vi "NewIndependentStage.vi"() -> ()   [LabVIEW 2020]
uses:
  StageOptions.ctl
  SettingCtrlOptions.ctl
  PosCtrlOptions.ctl
  libximc.lvlib
  <instrlib>/_niInstr/Basic Elements/v1/FPGA/niInstr Basic Elements v1 FPGA.lvlib
panel:
  out "Y Maximum":dbl=220.0
  out "X Max Stage":dbl=220.0 format="%#_13g"
  out "Move Step halved":dbl=1.0
  in  "Next Coordinate Index":i32
  out "Step Sizes":sgl[](array[numeric])
  out "IDs":i32[](array[numeric])
  out "Calibration":cluster{dbl, "MicrostepMode":u32}[](array[cluster])
  out "Serial nos":u32[](array[numeric])
  in  "EdgePt/nPixelMap":bool=TRUE
  out "Stage Status":T1
  in  "Machine Mode":T2(ring)=enum."Normal"
  in  "Close Stage":bool
  in  "Move Step":dbl=1.0
  in  "Start Stage":bool
  in  "Speed Control (mm/s)":sgl(slide)=1.0 min=0.1 scale=0.1..5.0
  out "Y Step Size":sgl format="%#_2g"
  out "X Step Size":sgl format="%#_2g"
  in  "Scan Mode":enum16{"Raster", "Serpentine"}(ring)
  out "Controller Open?":bool
  in  "Y Position Abs":dbl caption="Y Position"
  in  "X Position Abs":dbl caption="X Position"
  in  "Move to Start":bool
  in  "Stop Stage":bool
  in  "Outline":bool
  in  "Stop Motion":bool
  in  "Right":bool
  in  "Left":bool
  in  "Down":bool
  in  "Up":bool
  in  "AbsMove":bool
  out "Moving?":bool
  in  "Zero":bool
  out "Y Position":dbl format="%#.3g"
  out "X Position":dbl format="%#.3g"
  out "Stage Position":cluster{sgl[], sgl[]}(graph) caption="XY Graph - Dark"
  in  "X Start":sgl
  in  "X End":sgl=10.0
  in  "Y Start":sgl
  in  "Y End":sgl=8.0
  in  "Y Step Size":sgl=0.5
  in  "X Step Size":sgl=0.5
  out "Line Count":i32=6
  out "Pixel Count":i32=6
  out "Peripheral Coordis":sgl[][](array[numeric])=[[0.0, 0.0], [1.8, 0.0], [3.6, 0.0], [5.3999996, 0.0], [7.2, 0.0], [9.0, 0.0], [9.0, 2.0], [7.2, 2.0], [5.3999996, 2.0], [3.6, 2.0], [1.8, 2.0], [0.0, 2.0], [0.0, 4.0], [1.8, 4.0], [3.6, 4.0], [5.3999996, 4.0], [7.2, 4.0], [9.0, 4.0], [9.0, 6.0], [7.2, 6.0], [5.3999996, 6.0], [3.6, 6.0], [1.8, 6.0], [0.0, 6.0], [0.0, 8.0], [1.8, 8.0], [3.6, 8.0], [5.3999996, 8.0], [7.2, 8.0], [9.0, 8.0], [9.0, 10.0], [7.2, 10.0], [5.3999996, 10.0], [3.6, 10.0], [1.8, 10.0], [0.0, 10.0]]
  out "Coordinate Array":sgl[][](array[numeric])
  in  "Correction Table Path (Hidden)":path
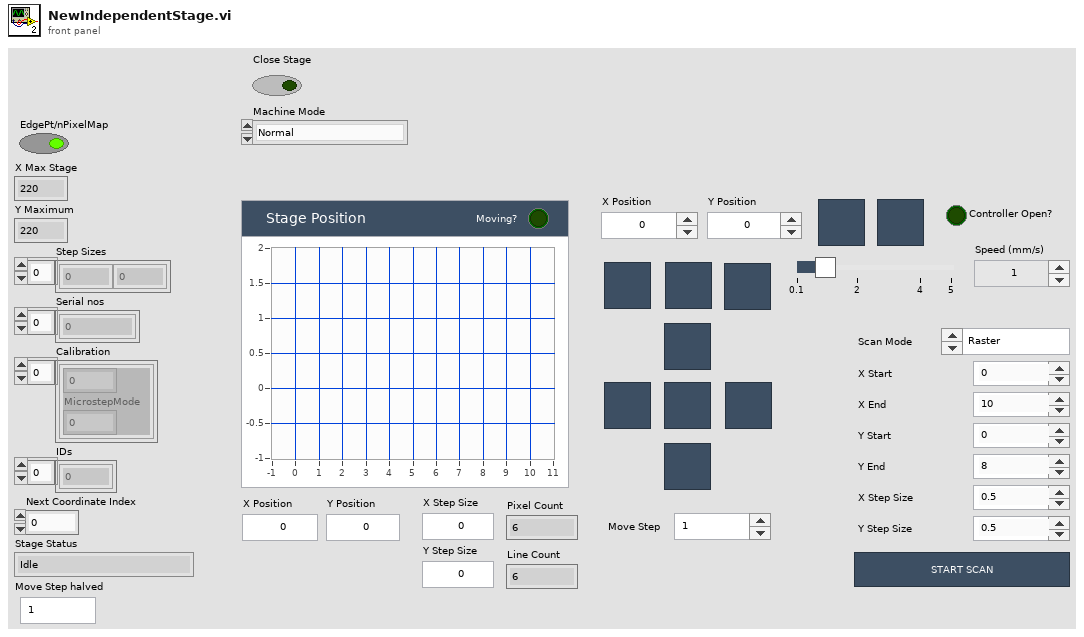
[diagram p1: front panel]
types:
  T1 = typedef "StageOptions.ctl" = enum16{"Idle", "Init", "Set Speed", "GenerateMotionPoints", "Scan_Start", "Scan_MoveNext", "Scan_SyncSet", "Scan_Get Pos", "Scan_Complete", "Cmd_MoveAbs", "Cmd_CloseControllers", "Cmd_MoveUp", "Cmd_MoveDown", "Cmd_MoveLeft", "Cmd_MoveRight", "Cmd_MoveStart", "Cmd_MoveZero", "Cmd_GetPos", "Cmd_Stop", "Sync_On", "Sync_Off", "Stop Motion", "CloseApplication"}
  T2 = enum16{"Scanning Mode", "Perimeter Mode", "Normal"}
  T3 = typedef "SettingCtrlOptions.ctl" = enum16{"Set X", "Set Y", "Set X and Y", "Get Settings", "None"}
  T4 = typedef "PosCtrlOptions.ctl" = enum16{"Move X", "Move Y", "Both X and Y", "Read Pos", "None"}
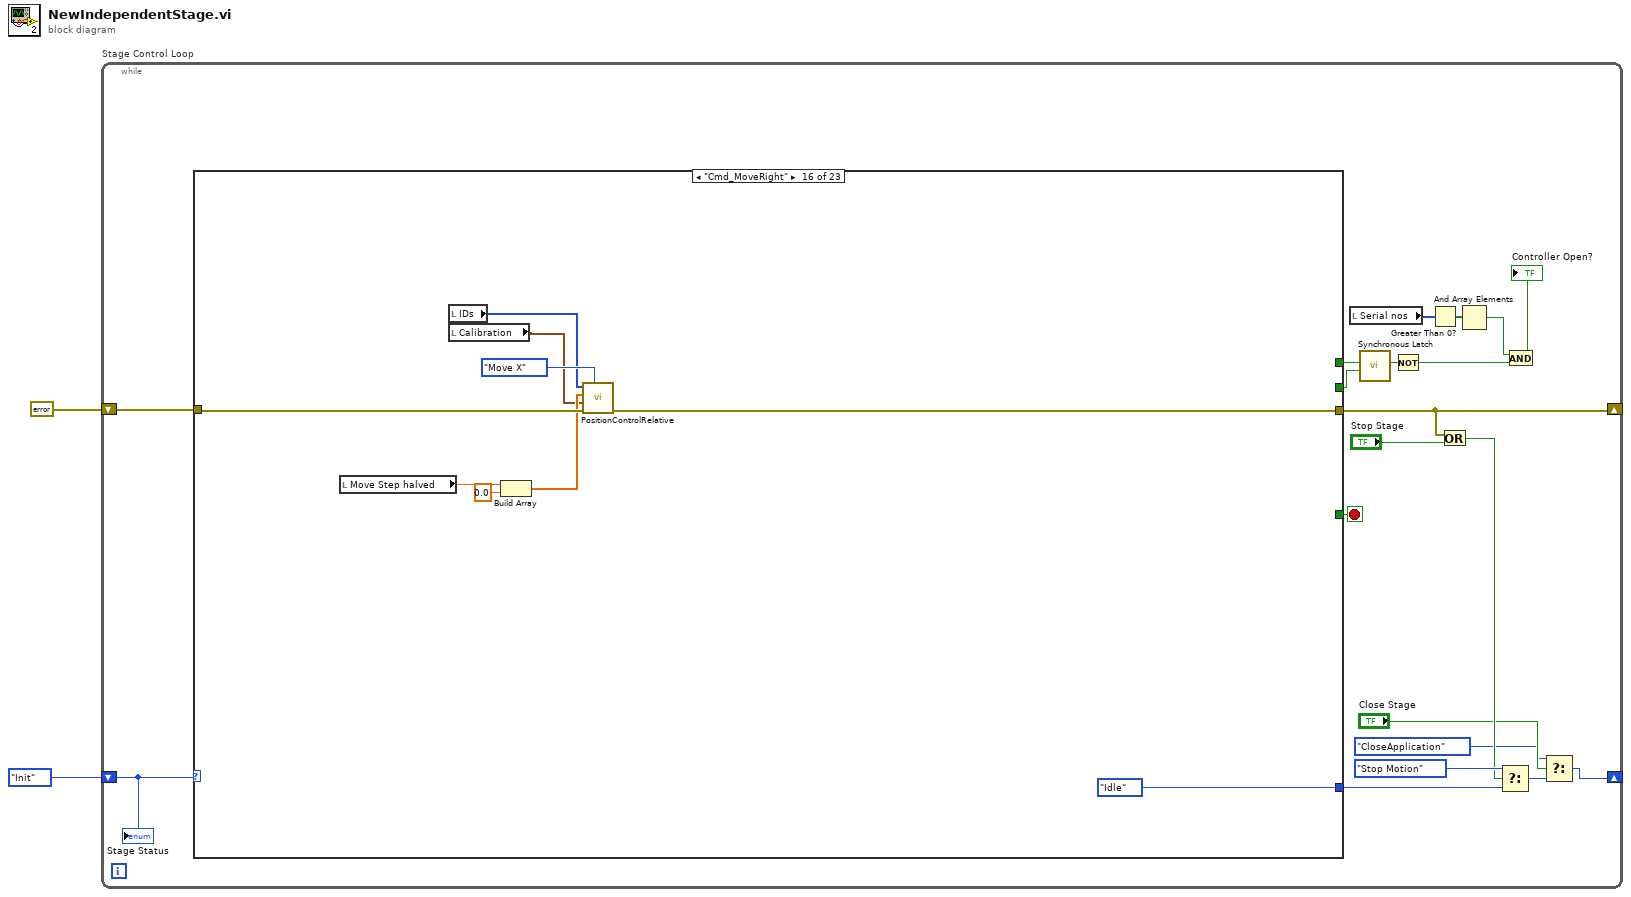
[diagram p0: block diagram]
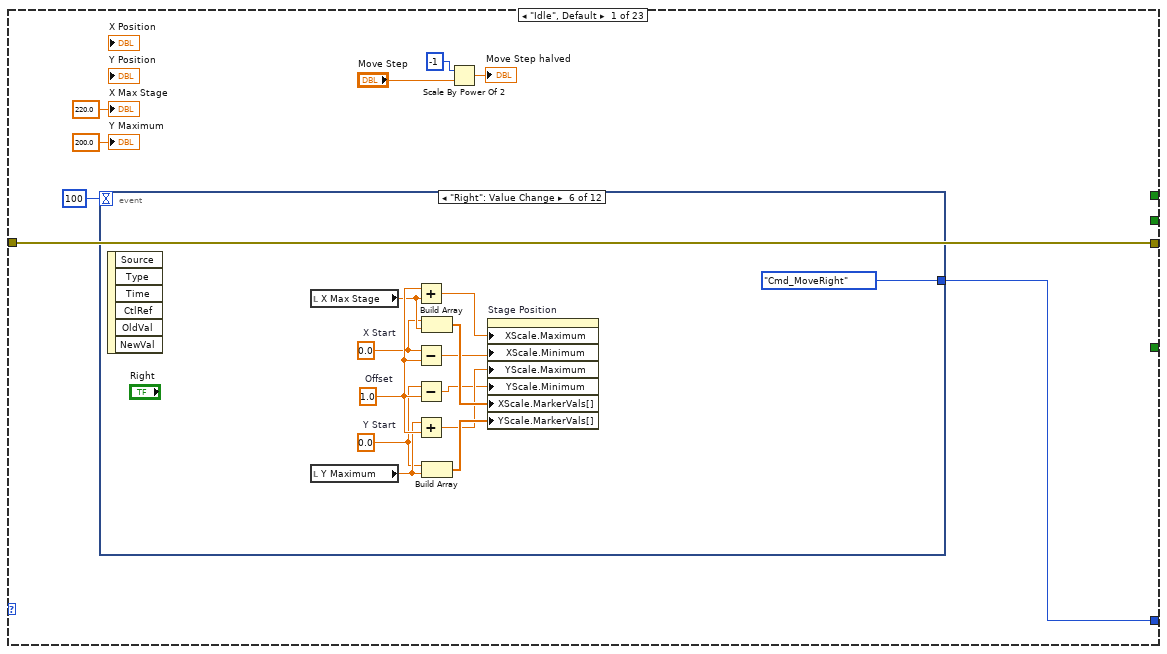
[diagram p2: hidden frame]
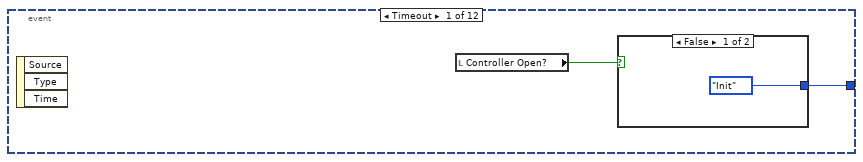
[diagram p3: hidden frame]
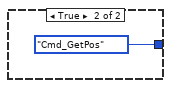
[diagram p4: hidden frame]
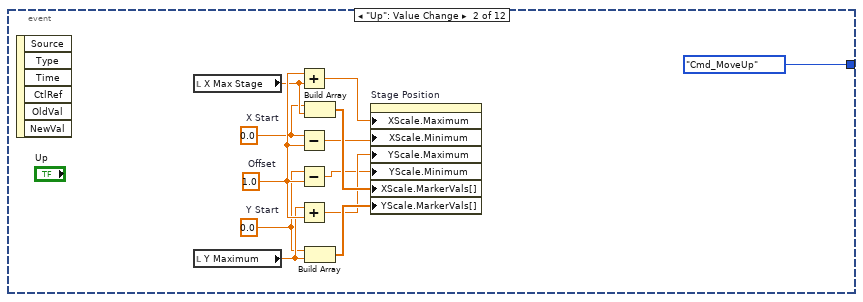
[diagram p5: hidden frame]
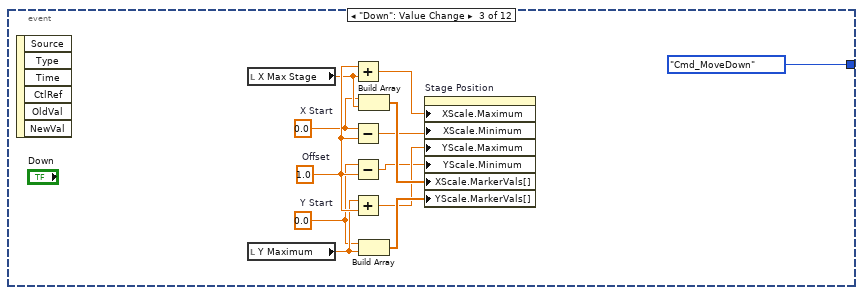
[diagram p6: hidden frame]
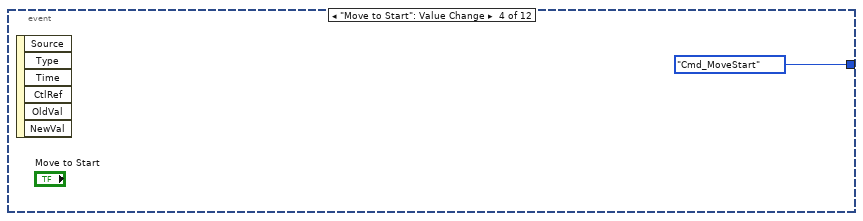
[diagram p7: hidden frame]
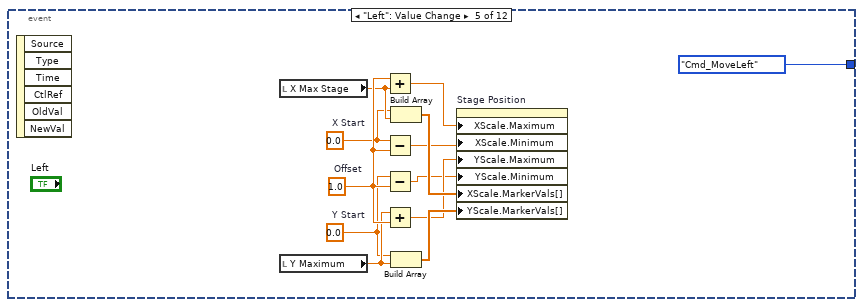
[diagram p8: hidden frame]
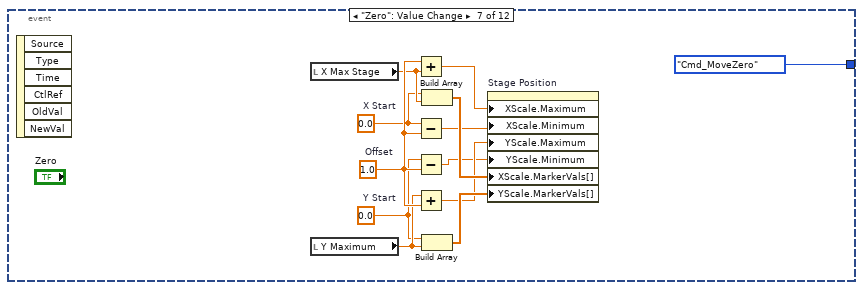
[diagram p9: hidden frame]
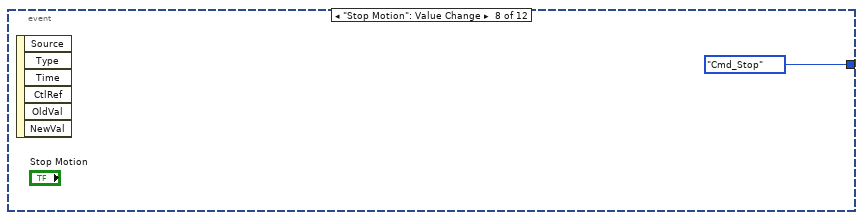
[diagram p10: hidden frame]
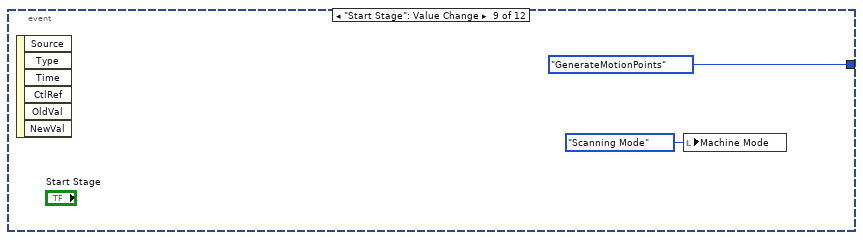
[diagram p11: hidden frame]
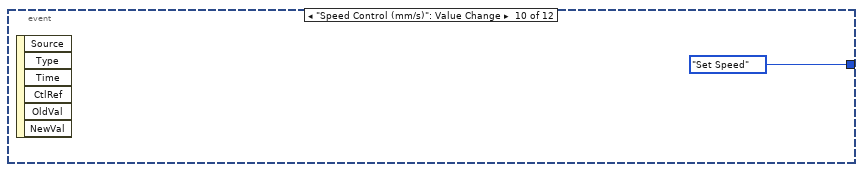
[diagram p12: hidden frame]
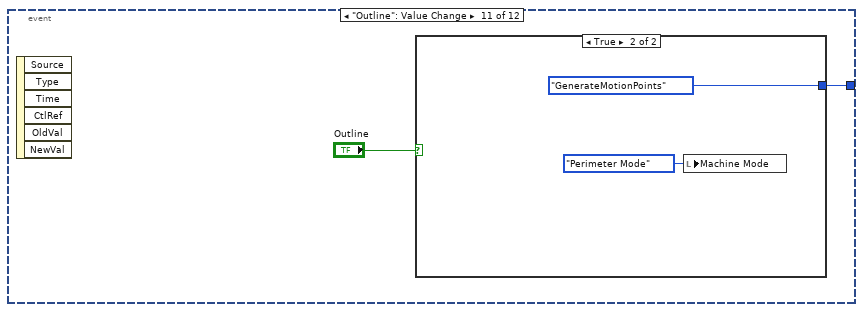
[diagram p13: hidden frame]
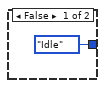
[diagram p14: hidden frame]
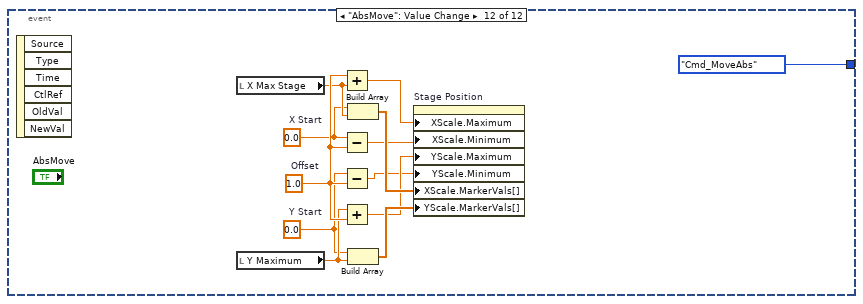
[diagram p15: hidden frame]
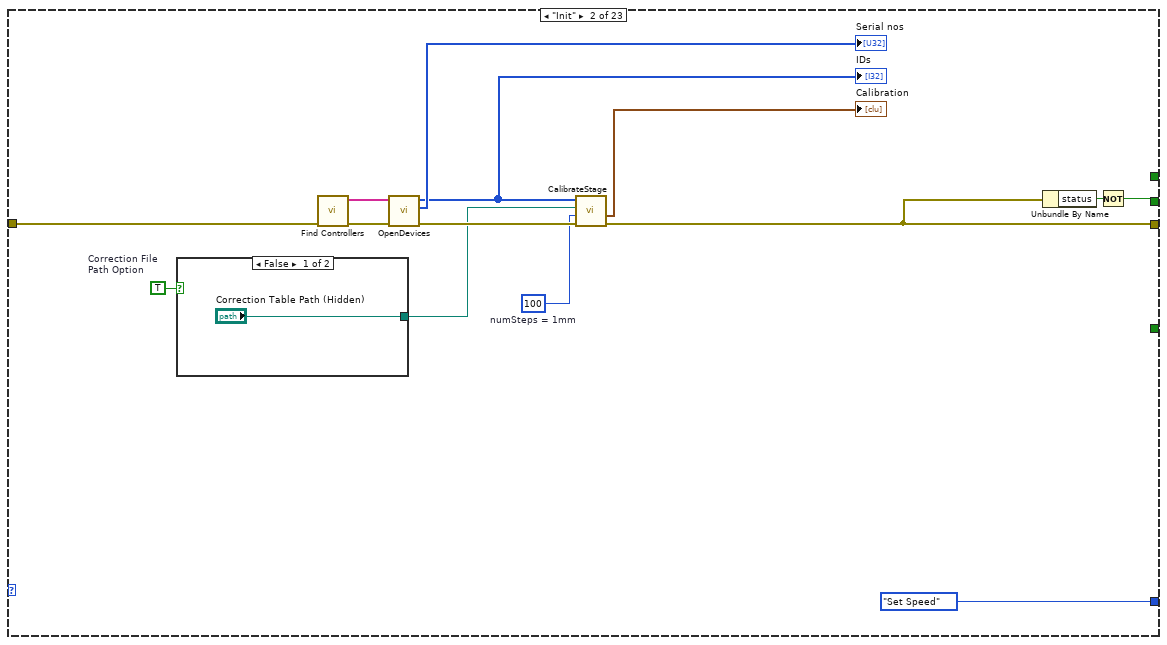
[diagram p16: hidden frame]
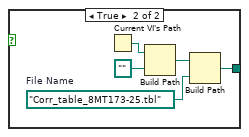
[diagram p17: hidden frame]
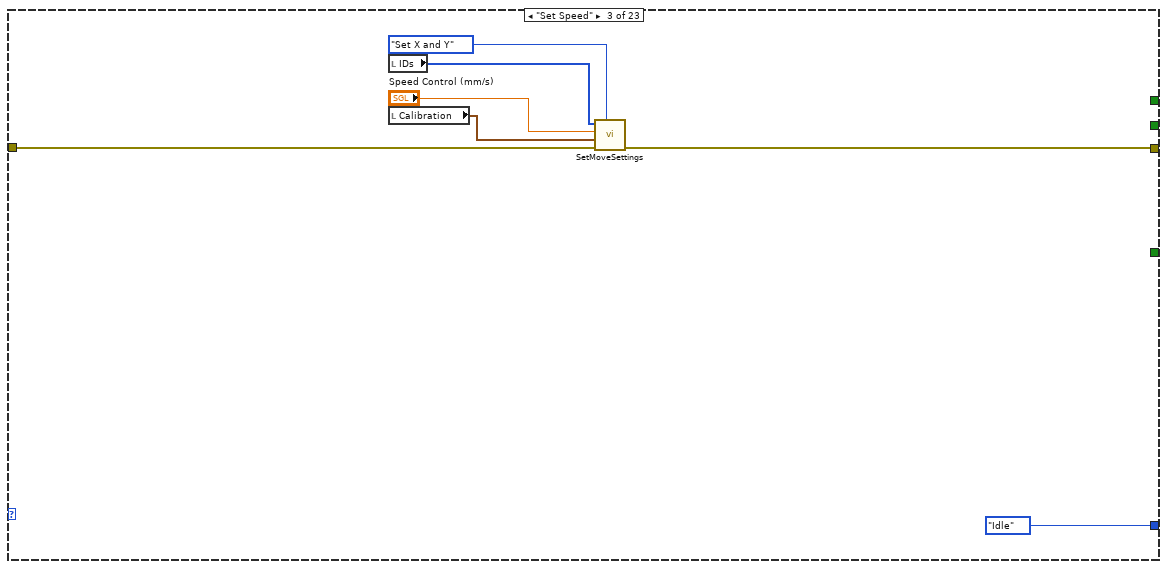
[diagram p18: hidden frame]
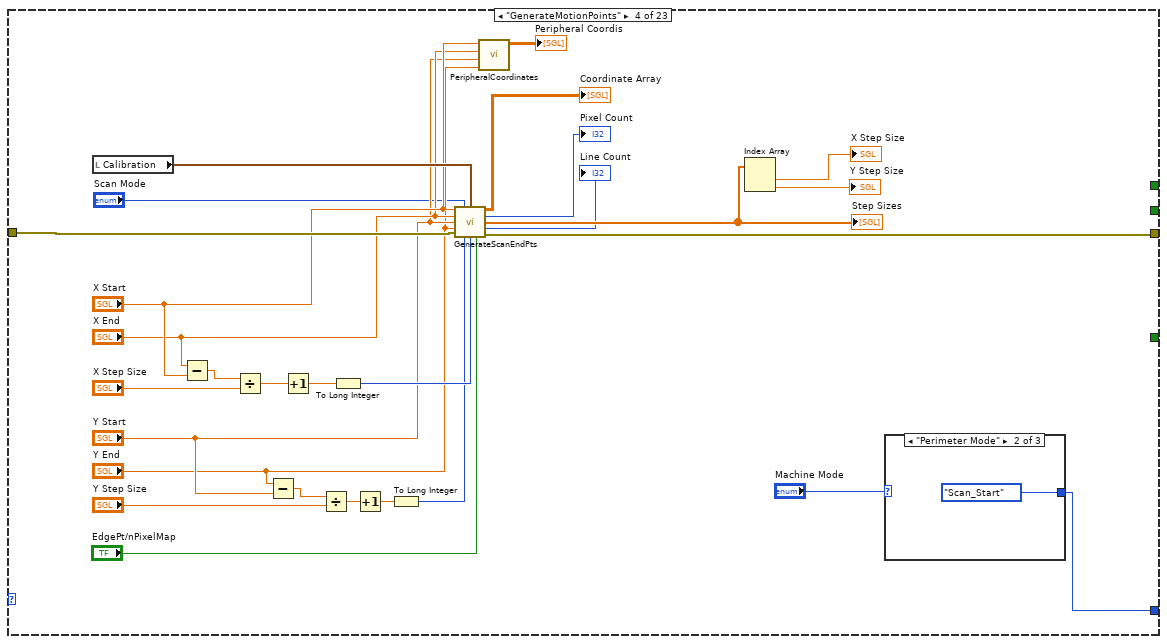
[diagram p19: hidden frame]
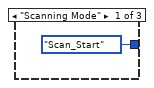
[diagram p20: hidden frame]
diagram:
  n1 = while "Stage Control Loop" {
    shift-right: [w11] -> _
    shift-left: StageOptions."Init" -> [w22]
    shift-right: [w19] -> _
    shift-left: errorcluster {"status"=FALSE, "code"=0, "source"=""} ("error out") -> [w20]
    stop <- w12 stop-if-true
    n2 = case shown="\"Cmd_MoveRight\"" w22 {
      tunnel: [w30 w117 w140 w171 w185 w217 w231 w244 w285 w294 w303 w310 w321 w331 w341 w350 w358 w373 w379 w390 w399 w406 w416] -> w19
      tunnel: w20 -> [w30 w124 w141 w170 w191 w218 w232 w245 w286 w295 w304 w309 w322 w332 w342 w351 w359 w374 w378 w391 w400 w405 w415]
      tunnel: [w29 StageOptions."Set Speed" StageOptions."Idle" w155 StageOptions."Scan_Get Pos" w206 StageOptions."Scan_MoveNext" w241 StageOptions."Idle" StageOptions."Idle" StageOptions."Idle" StageOptions."Idle" StageOptions."Idle" StageOptions."Idle" StageOptions."Idle" StageOptions."Idle" StageOptions."Idle" StageOptions."Idle" StageOptions."Idle" StageOptions."Idle" StageOptions."Idle" StageOptions."Idle" StageOptions."Idle"] -> w17
      tunnel: [_ _ _ _ _ _ _ _ _ _ _ _ _ _ _ _ _ _ _ _ _ w402 w411] -> w15
      tunnel: [_ w118 _ _ _ _ _ _ _ _ _ _ _ _ _ _ _ _ _ _ _ _ _] -> w13
      tunnel: [_ _ _ _ _ _ _ _ _ _ _ _ _ _ _ _ _ _ _ _ _ _ w411] -> w12
      frame "Idle", Default {
        n3 = event shown="[5] \"Right\": Value Change" {
          selector: _ -> [_ _ _ _ _ _ _ _ _ _ _ _]
          dyn-events: _ -> [_ _ _ _ _ _ _ _ _ _ _ _]
          timeout: 100 -> [_ _ _ _ _ _ _ _ _ _ _ _]
          tunnel: [w31 StageOptions."Cmd_MoveUp" StageOptions."Cmd_MoveDown" StageOptions."Cmd_MoveStart" StageOptions."Cmd_MoveLeft" StageOptions."Cmd_MoveRight" StageOptions."Cmd_MoveZero" StageOptions."Cmd_Stop" StageOptions."GenerateMotionPoints" StageOptions."Set Speed" w101 StageOptions."Cmd_MoveAbs"] -> w29
          event Timeout {
            n4 = event-data() -> ()  [unwired: 1 in, 3 out]
            n5 = local read "Controller Open?"() -> (w32:bool)
            n6 = case shown="False" w32 {
              tunnel: [StageOptions."Init" StageOptions."Cmd_GetPos"] -> w31
              frame False {
              }
              frame True {
              }
            }
          }
          event "Up": Value Change {
            w35 = 0.0  # Y Start
            w37 = sgl 0.0  # X Start
            w40 = 1.0  # Offset
            n7 = event-data() -> ()  [unwired: 1 in, 6 out]
            n8 = local read "X Max Stage"() -> (w38:dbl)
            n9 = local read "Y Maximum"() -> (w36:dbl)
            n10 = Add(x=w40, y=w38) -> (x+y=w42:dbl)
            n11 = Subtract(x=w37, y=w40) -> (x-y=w43:dbl)
            n12 = Subtract(x=w35, y=w40) -> (x-y=w39:dbl)
            n13 = Add(x=w36, y=w40) -> (x+y=w41:dbl)
            n14 = Build Array(w37, w38) -> (w45:dbl[])
            n15 = Build Array(w35, w36) -> (w44:dbl[])
            n16 = property on="Stage Position" class="XYGraph (strict)"("XScale.Maximum"=w42, "XScale.Minimum"=w43, "YScale.Maximum"=w41, "YScale.Minimum"=w39, "XScale.MarkerVals[]"=w45, "YScale.MarkerVals[]"=w44) -> ()  [unwired: 2 in, 2 out]
          }
          event "Down": Value Change {
            w47 = 0.0  # Y Start
            w49 = sgl 0.0  # X Start
            w52 = 1.0  # Offset
            n17 = event-data() -> ()  [unwired: 1 in, 6 out]
            n18 = local read "X Max Stage"() -> (w50:dbl)
            n19 = local read "Y Maximum"() -> (w48:dbl)
            n20 = Add(x=w52, y=w50) -> (x+y=w54:dbl)
            n21 = Subtract(x=w49, y=w52) -> (x-y=w55:dbl)
            n22 = Subtract(x=w47, y=w52) -> (x-y=w51:dbl)
            n23 = Add(x=w48, y=w52) -> (x+y=w53:dbl)
            n24 = Build Array(w49, w50) -> (w57:dbl[])
            n25 = Build Array(w47, w48) -> (w56:dbl[])
            n26 = property on="Stage Position" class="XYGraph (strict)"("XScale.Maximum"=w54, "XScale.Minimum"=w55, "YScale.Maximum"=w53, "YScale.Minimum"=w51, "XScale.MarkerVals[]"=w57, "YScale.MarkerVals[]"=w56) -> ()  [unwired: 2 in, 2 out]
          }
          event "Move to Start": Value Change {
            n27 = event-data() -> ()  [unwired: 1 in, 6 out]
          }
          event "Left": Value Change {
            w60 = 0.0  # Y Start
            w62 = sgl 0.0  # X Start
            w65 = 1.0  # Offset
            n28 = event-data() -> ()  [unwired: 1 in, 6 out]
            n29 = local read "X Max Stage"() -> (w63:dbl)
            n30 = local read "Y Maximum"() -> (w61:dbl)
            n31 = Add(x=w65, y=w63) -> (x+y=w67:dbl)
            n32 = Subtract(x=w62, y=w65) -> (x-y=w68:dbl)
            n33 = Subtract(x=w60, y=w65) -> (x-y=w64:dbl)
            n34 = Add(x=w61, y=w65) -> (x+y=w66:dbl)
            n35 = Build Array(w62, w63) -> (w70:dbl[])
            n36 = Build Array(w60, w61) -> (w69:dbl[])
            n37 = property on="Stage Position" class="XYGraph (strict)"("XScale.Maximum"=w67, "XScale.Minimum"=w68, "YScale.Maximum"=w66, "YScale.Minimum"=w64, "XScale.MarkerVals[]"=w70, "YScale.MarkerVals[]"=w69) -> ()  [unwired: 2 in, 2 out]
          }
          event "Right": Value Change {
            w72 = 0.0  # Y Start
            w74 = sgl 0.0  # X Start
            w77 = 1.0  # Offset
            n38 = event-data() -> ()  [unwired: 1 in, 6 out]
            n39 = local read "X Max Stage"() -> (w75:dbl)
            n40 = local read "Y Maximum"() -> (w73:dbl)
            n41 = Add(x=w77, y=w75) -> (x+y=w79:dbl)
            n42 = Subtract(x=w74, y=w77) -> (x-y=w80:dbl)
            n43 = Subtract(x=w72, y=w77) -> (x-y=w76:dbl)
            n44 = Add(x=w73, y=w77) -> (x+y=w78:dbl)
            n45 = Build Array(w74, w75) -> (w82:dbl[])
            n46 = Build Array(w72, w73) -> (w81:dbl[])
            n47 = property on="Stage Position" class="XYGraph (strict)"("XScale.Maximum"=w79, "XScale.Minimum"=w80, "YScale.Maximum"=w78, "YScale.Minimum"=w76, "XScale.MarkerVals[]"=w82, "YScale.MarkerVals[]"=w81) -> ()  [unwired: 2 in, 2 out]
          }
          event "Zero": Value Change {
            w84 = 0.0  # Y Start
            w86 = sgl 0.0  # X Start
            w89 = 1.0  # Offset
            n48 = event-data() -> ()  [unwired: 1 in, 6 out]
            n49 = local read "X Max Stage"() -> (w87:dbl)
            n50 = local read "Y Maximum"() -> (w85:dbl)
            n51 = Add(x=w89, y=w87) -> (x+y=w91:dbl)
            n52 = Subtract(x=w86, y=w89) -> (x-y=w92:dbl)
            n53 = Subtract(x=w84, y=w89) -> (x-y=w88:dbl)
            n54 = Add(x=w85, y=w89) -> (x+y=w90:dbl)
            n55 = Build Array(w86, w87) -> (w94:dbl[])
            n56 = Build Array(w84, w85) -> (w93:dbl[])
            n57 = property on="Stage Position" class="XYGraph (strict)"("XScale.Maximum"=w91, "XScale.Minimum"=w92, "YScale.Maximum"=w90, "YScale.Minimum"=w88, "XScale.MarkerVals[]"=w94, "YScale.MarkerVals[]"=w93) -> ()  [unwired: 2 in, 2 out]
          }
          event "Stop Motion": Value Change {
            n58 = event-data() -> ()  [unwired: 1 in, 6 out]
          }
          event "Start Stage": Value Change {
            n59 = event-data() -> ()  [unwired: 1 in, 6 out]
            n60 = local write "Machine Mode"(T2."Scanning Mode" ("Machine Mode")) -> ()
          }
          event "Speed Control (mm/s)": Value Change {
            n61 = event-data() -> ()  [unwired: 1 in, 6 out]
          }
          event "Outline": Value Change {
            n62 = event-data() -> ()  [unwired: 1 in, 6 out]
            n63 = case shown="True" "Outline" {
              tunnel: [StageOptions."Idle" StageOptions."GenerateMotionPoints"] -> w101
              frame False {
              }
              frame True {
                n64 = local write "Machine Mode"(T2."Perimeter Mode" ("Machine Mode")) -> ()
              }
            }
          }
          event "AbsMove": Value Change {
            w105 = 0.0  # Y Start
            w107 = sgl 0.0  # X Start
            w110 = 1.0  # Offset
            n65 = event-data() -> ()  [unwired: 1 in, 6 out]
            n66 = local read "X Max Stage"() -> (w108:dbl)
            n67 = local read "Y Maximum"() -> (w106:dbl)
            n68 = Add(x=w110, y=w108) -> (x+y=w112:dbl)
            n69 = Subtract(x=w107, y=w110) -> (x-y=w113:dbl)
            n70 = Subtract(x=w105, y=w110) -> (x-y=w109:dbl)
            n71 = Add(x=w106, y=w110) -> (x+y=w111:dbl)
            n72 = Build Array(w107, w108) -> (w115:dbl[])
            n73 = Build Array(w105, w106) -> (w114:dbl[])
            n74 = property on="Stage Position" class="XYGraph (strict)"("XScale.Maximum"=w112, "XScale.Minimum"=w113, "YScale.Maximum"=w111, "YScale.Minimum"=w109, "XScale.MarkerVals[]"=w115, "YScale.MarkerVals[]"=w114) -> ()  [unwired: 2 in, 2 out]
          }
        }
        n75 = Scale By Power Of 2(n=i16 -1, x="Move Step") -> (x*2^n=→"Move Step halved":dbl)
        "X Max Stage" <- 220.0 ("X Max Stage")
        "Y Maximum" <- 200.0 ("Y Maximum")
      }
      frame "Init" {
        w125 = 100  # numSteps = 1mm
        w126 = TRUE  # Correction File Path Option
        n76 = case shown="False" w126 {
          tunnel: ["Correction Table Path (Hidden)" w132] -> w127
          frame False {
          }
          frame True {
            w133 = path "Corr_table_8MT173-25.tbl"  # File Name
            n77 = Current VI's Path() -> (path=w135:path)
            n78 = Build Path(base path=w135, name or relative path=path "") -> (appended path=w134:path)
            n79 = Build Path(base path=w134, name or relative path=w133) -> (appended path=w132:path)
          }
        }
        n80 = call "Find Controllers.vi"("error in (no error)"=w124) -> ("error out"=w129:errorcluster, "Names"=w130:string[])  [unwired: 8 in, 1 out]
        n81 = call "OpenDevices.vi"("error In"=w129, "Names"=w130) -> ("error out"=w128:errorcluster, "Serial nos"=→"Serial nos":u32[], "IDs"=w122:i32[])  [unwired: 6 in]
        "IDs" <- w122
        n82 = call "CalibrateStage.vi"("error in (no error)"=w128, "numSteps = 1mm"=w125, "Correction Table Path"=w127, "IDs"=w122) -> ("error out"=w117:errorcluster, "Calibration"=→"Calibration":cluster{dbl, "MicrostepMode":u32}[])  [unwired: 2 in, 4 out]
        n83 = Unbundle By Name(w117) -> ("status"=w119:bool)
        n84 = Not(x=w119) -> (.not. x?=w118:bool)
      }
      frame "Set Speed" {
        n85 = local read "IDs"() -> (w139:i32[])
        n86 = local read "Calibration"() -> (w138:cluster{dbl, "MicrostepMode":u32}[])
        n87 = call "SetMoveSettings.vi"("Mode"=SettingCtrlOptions."Set X and Y", "error in (no error)"=w141, "Calibration"=w138, "Speed"="Speed Control (mm/s)", "IDs"=w139) -> ("error out"=w140:errorcluster)  [unwired: 4 in, 2 out]
      }
      frame "GenerateMotionPoints" {
        n88 = local read "Calibration"() -> (w161:cluster{dbl, "MicrostepMode":u32}[])
        n89 = Subtract(x="X End", y="X Start") -> (x-y=w148:sgl)
        n90 = Divide(x=w148, y="X Step Size") -> (x/y=w166:sgl)
        n91 = Subtract(x="Y End", y="Y Start") -> (x-y=w146:sgl)
        n92 = Increment(x=w166) -> (x+1=w151:sgl)
        n93 = Divide(x=w146, y="Y Step Size") -> (x/y=w163:sgl)
        n94 = To Long Integer(number=w151) -> (32bit integer=w165:i32)
        n95 = Increment(x=w163) -> (x+1=w150:sgl)
        n96 = To Long Integer(number=w150) -> (32bit integer=w162:i32)
        n97 = call "GenerateScanEndPts.vi"("X Start"="X Start", "Mode"="Scan Mode", "Calibration In"=w161, "X End"="X End", "Y Start"="Y Start", "Y End"="Y End", "error in"=w170, "Line Count"=w162, "Pixel Count"=w165, "EdgePt/nPixelMap"="EdgePt/nPixelMap") -> ("Coordinate Array"=→"Coordinate Array":sgl[][], "X Pixel Count"=→"Pixel Count":i32, "Step Sizes"=w152:sgl[], "Y Pixel Count"=→"Line Count":i32, "error out"=w171:errorcluster)  [unwired: 1 in]
        "Step Sizes" <- w152
        n98 = call "PeripheralCoordinates.vi"("Y End"="Y End", "Y Start"="Y Start", "X End"="X End", "X Start"="X Start") -> ("Coordinate Array"=→"Peripheral Coordis":sgl[][])  [unwired: 7 in]
        n99 = Index Array(array=w152) -> (element #1=→"X Step Size":sgl, element #2=→"Y Step Size":sgl)  [unwired: 2 in]
        n100 = case shown="\"Perimeter Mode\"" "Machine Mode" {
          tunnel: [StageOptions."Scan_Start" StageOptions."Scan_Start" StageOptions."Idle"] -> w155
          frame "Scanning Mode" {
          }
          frame "Perimeter Mode" {
          }
          frame "Normal", Default {
          }
        }
      }
      frame "Scan_Start" {
        w188 = 0.0 ("element")
        w197 = 1.0  # Offset
        # "Draw Markers To Indicate the Scan Area"
        n101 = property on="X End" class="DigNum (strict)"() -> ("Value"=w196:sgl)  [unwired: 2 in, 2 out]
        n102 = property on="X Start" class="DigNum (strict)"() -> ("Value"=w195:sgl)  [unwired: 2 in, 2 out]
        n103 = property on="Y End" class="DigNum (strict)"() -> ("Value"=w192:sgl)  [unwired: 2 in, 2 out]
        n104 = property on="Y Start" class="DigNum (strict)"() -> ("Value"=w194:sgl)  [unwired: 2 in, 2 out]
        n105 = Add(x=w197, y=w196) -> (x+y=w199:dbl)
        n106 = Subtract(x=w195, y=w197) -> (x-y=w200:dbl)
        n107 = Add(x=w192, y=w197) -> (x+y=w198:dbl)
        n108 = Subtract(x=w194, y=w197) -> (x-y=w193:dbl)
        n109 = Build Array(w195, w196) -> (w202:sgl[])
        n110 = Build Array(w194, w192) -> (w201:sgl[])
        n111 = property on="Stage Position" class="XYGraph (strict)"(error in=w191, "XScale.Maximum"=w199, "XScale.Minimum"=w200, "YScale.Maximum"=w198, "YScale.Minimum"=w193, "XScale.MarkerVals[]"=w202, "YScale.MarkerVals[]"=w201) -> (error out=w177:errorcluster)  [unwired: 1 in, 1 out]
        n112 = local read "EdgePt/nPixelMap"() -> (w181:bool)
        n113 = local read "IDs"() -> (w184:i32[])
        n114 = local read "Step Sizes"() -> (w182:sgl[])
        n115 = local read "Calibration"() -> (w183:cluster{dbl, "MicrostepMode":u32}[])
        n116 = call "SetSyncSettings.vi"("Periodic/nPointScan"=w181, "X SyncOut Enabled"=FALSE, "Y SyncOut Enabled"=FALSE, "error in (no error)"=w177, "Calibration"=w183, "Step Sizes(mm)"=w182, "IDs"=w184) -> ("error out"=w178:errorcluster)  [unwired: 3 in, 1 out]
        n117 = local write "Next Coordinate Index"(0 ("Next Coordinate Index")) -> ()
        n118 = local read "IDs"() -> (w186:i32[])
        n119 = local read "Calibration"() -> (w187:cluster{dbl, "MicrostepMode":u32}[])
        n120 = Build Array(w188, w188) -> (w189:dbl[])
        n121 = call "PositionControlRelative.vi"("Mode"=PosCtrlOptions."Both X and Y", "error in (no error)"=w178, "Calibration"=w187, "Move to"=w189, "IDs"=w186) -> ("error out"=w185:errorcluster)  [unwired: 4 in, 2 out]
      }
      frame "Scan_Get Pos" {
        n122 = local read "IDs"() -> (w215:i32[])
        n123 = local read "Calibration"() -> (w216:cluster{dbl, "MicrostepMode":u32}[])
        n124 = call "PositionControl.vi"("Mode"=PosCtrlOptions."Read Pos", "error in (no error)"=w218, "Calibration"=w216, "IDs"=w215) -> ("error out"=w217:errorcluster, "Moving?"=w205:bool, "Position"=w208:sgl[])  [unwired: 4 in, 1 out]
        n125 = local write "Moving?"(w205) -> ()
        n126 = Index Array(array=w208, index #1=0 ("index"), index #2=1 ("index")) -> (element #1=w212:sgl, element #2=w211:sgl)
        n127 = local write "X Position"(w212) -> ()
        n128 = local write "Y Position"(w211) -> ()
        n129 = Build Array(w212) -> (w213:sgl[])
        n130 = Build Array(w211) -> (w214:sgl[])
        n131 = Bundle(w213, w214) -> (w207:cluster{sgl[], sgl[]})  [unwired: 1 in]
        n132 = local write "Stage Position"(w207) -> ()
        n133 = Select(t=StageOptions."Scan_Get Pos", s=w205, f=StageOptions."Scan_SyncSet") -> (s? t:f=w206:T1)
      }
      frame "Scan_SyncSet" {
        n134 = local read "EdgePt/nPixelMap"() -> (w221:bool)
        n135 = local read "IDs"() -> (w229:i32[])
        n136 = local read "Step Sizes"() -> (w227:sgl[])
        n137 = local read "Calibration"() -> (w228:cluster{dbl, "MicrostepMode":u32}[])
        n138 = Quotient & Remainder(x="Next Coordinate Index", y=2) -> (x-y*floor(x/y)=w224:i32)  [unwired: 1 out]
        n139 = Not Equal To 0?(x=w224) -> (x != 0?=w222:bool)
        n140 = Compound Arithmetic op=OR(invert w221, w222) -> (w223:bool)
        n141 = call "SetSyncSettings.vi"("Periodic/nPointScan"=w221, "X SyncOut Enabled"=w223, "Y SyncOut Enabled"=FALSE, "error in (no error)"=w232, "Calibration"=w228, "Step Sizes(mm)"=w227, "IDs"=w229) -> ("error out"=w231:errorcluster)  [unwired: 3 in, 1 out]
      }
      frame "Scan_MoveNext" {
        n142 = flat-sequence {
          tunnel: w245 -> [w248]
          tunnel: [w248] -> w236
          tunnel: [w247] -> w235
          tunnel: [w246] -> w233
          tunnel: [w256] -> w243
          tunnel: [w253] -> w242
          tunnel: [w252] -> w238
          tunnel: w236 -> [w257]
          tunnel: w235 -> [w252]
          tunnel: [w251] -> w234
          tunnel: w233 -> [w251]
          tunnel: [w267] -> w237
          tunnel: [w268] -> w244
          tunnel: w234 -> [w260]
          tunnel: w238 -> [w264]
          tunnel: w242 -> [w265]
          tunnel: w243 -> [w268]
          frame #0 {
            n143 = local read "Machine Mode"() -> (w246:T2)
            n144 = case shown="\"Perimeter Mode\"" w246 {
              tunnel: [w249 w250] -> w247
              frame "Scanning Mode", Default {
                n145 = local read "Coordinate Array"() -> (w249:sgl[][])
              }
              frame "Perimeter Mode" {
                n146 = local read "Peripheral Coordis"() -> (w250:sgl[][])
              }
            }
          }
          frame #1 {
            n147 = local read "IDs"() -> (w255:i32[])
            n148 = local read "Next Coordinate Index"() -> (w253:i32)
            n149 = local read "Calibration"() -> (w254:cluster{dbl, "MicrostepMode":u32}[])
            n150 = Index Array(array=w252, index (row)=w253) -> (element=w258:sgl[])  [unwired: 1 in]
            n151 = call "PositionControl.vi"("Mode"=PosCtrlOptions."Both X and Y", "error in (no error)"=w257, "Calibration"=w254, "Move to"=w258, "IDs"=w255) -> ("error out"=w256:errorcluster)  [unwired: 3 in, 3 out]
          }
          frame #2 {
            n152 = Matrix Size(0:w264) -> (1:w263:i32)  [unwired: 1 out]
            n153 = Increment(x=w265) -> (x+1=w261:i32)
            n154 = Greater?(x=w261, y=w263) -> (0:w262:bool)
            n155 = case shown="True" w262 {
              selector: w262 -> [w269 _]
              tunnel: w261 -> [w270 w273]
              tunnel: [w270 w272] -> w266
              tunnel: [w269 w271] -> w267
              tunnel: w260 -> [_ w274]
              frame False {
              }
              frame True {
                n156 = case shown="\"Scanning Mode\", Default" w274 {
                  tunnel: w273 -> [w276 _]
                  tunnel: [w276 0] -> w272
                  tunnel: [TRUE ("x > y?") w278] -> w271
                  frame "Scanning Mode", Default {
                  }
                  frame "Perimeter Mode" {
                    n157 = local read "Outline"() -> (w279:bool)
                    n158 = Not(x=w279) -> (.not. x?=w278:bool)
                  }
                }
              }
            }
            n159 = local write "Next Coordinate Index"(w266) -> ()
          }
        }
        n160 = Select(t=StageOptions."Scan_Complete", s=w237, f=StageOptions."Scan_Get Pos") -> (s? t:f=w241:T1)
      }
      frame "Scan_Complete" {
        w283 = 0.0 ("element")
        n161 = local read "IDs"() -> (w281:i32[])
        n162 = local read "Calibration"() -> (w282:cluster{dbl, "MicrostepMode":u32}[])
        n163 = Build Array(w283, w283) -> (w284:dbl[])
        n164 = call "PositionControl.vi"("Mode"=PosCtrlOptions."Both X and Y", "error in (no error)"=w286, "Calibration"=w282, "Move to"=w284, "IDs"=w281) -> ("error out"=w285:errorcluster)  [unwired: 3 in, 3 out]
      }
      frame "Cmd_MoveAbs" {
        n165 = local read "IDs"() -> (w293:i32[])
        n166 = local read "Calibration"() -> (w292:cluster{dbl, "MicrostepMode":u32}[])
        n167 = Build Array("X Position Abs", "Y Position Abs") -> (w291:dbl[])
        n168 = call "PositionControl.vi"("Mode"=PosCtrlOptions."Both X and Y", "error in (no error)"=w295, "Calibration"=w292, "Move to"=w291, "IDs"=w293) -> ("error out"=w294:errorcluster)  [unwired: 3 in, 3 out]
      }
      frame "Cmd_MoveStart" {
        n169 = local read "X Start"() -> (w298:sgl)
        n170 = local read "Y Start"() -> (w297:sgl)
        n171 = local read "IDs"() -> (w302:i32[])
        n172 = local read "Calibration"() -> (w301:cluster{dbl, "MicrostepMode":u32}[])
        n173 = Build Array(w298, w297) -> (w300:sgl[])
        n174 = call "PositionControl.vi"("Mode"=PosCtrlOptions."Both X and Y", "error in (no error)"=w304, "Calibration"=w301, "Move to"=w300, "IDs"=w302) -> ("error out"=w303:errorcluster)  [unwired: 3 in, 3 out]
      }
      frame "Cmd_CloseControllers" {
        n175 = local read "IDs"() -> (w307:i32[])
        n176 = for {
          shift-right: [w314] -> w311
          shift-left: w309 -> [w313]
          tunnel: w307 -> [w312] mode=indexing
          n177 = call "command stop.vi"("error in (no error)"=w313, "id"=w312) -> ("error out"=w314:errorcluster)  [unwired: 8 in, 1 out]
        }
        n178 = call "CloseDevices.vi"("error in (no error)"=w311, "Close"=TRUE, "Ids"=w307) -> ("error out"=w310:errorcluster)  [unwired: 8 in]
      }
      frame "Cmd_MoveUp" {
        n179 = local read "Move Step halved"() -> (w318:dbl)
        n180 = local read "IDs"() -> (w317:i32[])
        n181 = local read "Calibration"() -> (w316:cluster{dbl, "MicrostepMode":u32}[])
        n182 = Build Array(0.0 ("element"), w318) -> (w320:dbl[])
        n183 = call "PositionControlRelative.vi"("Mode"=PosCtrlOptions."Move Y", "error in (no error)"=w322, "Calibration"=w316, "Move to"=w320, "IDs"=w317) -> ("error out"=w321:errorcluster)  [unwired: 4 in, 2 out]
      }
      frame "Cmd_MoveDown" {
        n184 = local read "Move Step halved"() -> (w328:dbl)
        n185 = local read "IDs"() -> (w326:i32[])
        n186 = local read "Calibration"() -> (w325:cluster{dbl, "MicrostepMode":u32}[])
        n187 = Negate(x=w328) -> (-x=w327:dbl)
        n188 = Build Array(0.0 ("element"), w327) -> (w330:dbl[])
        n189 = call "PositionControlRelative.vi"("Mode"=PosCtrlOptions."Move Y", "error in (no error)"=w332, "Calibration"=w325, "Move to"=w330, "IDs"=w326) -> ("error out"=w331:errorcluster)  [unwired: 4 in, 2 out]
      }
      frame "Cmd_MoveLeft" {
        n190 = local read "Move Step halved"() -> (w339:dbl)
        n191 = local read "IDs"() -> (w335:i32[])
        n192 = local read "Calibration"() -> (w336:cluster{dbl, "MicrostepMode":u32}[])
        n193 = Negate(x=w339) -> (-x=w338:dbl)
        n194 = Build Array(w338, 0.0 ("element")) -> (w340:dbl[])
        n195 = call "PositionControlRelative.vi"("Mode"=PosCtrlOptions."Move X", "error in (no error)"=w342, "Calibration"=w336, "Move to"=w340, "IDs"=w335) -> ("error out"=w341:errorcluster)  [unwired: 4 in, 2 out]
      }
      frame "Cmd_MoveRight" {
        n196 = local read "Move Step halved"() -> (w348:dbl)
        n197 = local read "IDs"() -> (w346:i32[])
        n198 = local read "Calibration"() -> (w345:cluster{dbl, "MicrostepMode":u32}[])
        n199 = Build Array(w348, 0.0 ("element")) -> (w349:dbl[])
        n200 = call "PositionControlRelative.vi"("Mode"=PosCtrlOptions."Move X", "error in (no error)"=w351, "Calibration"=w345, "Move to"=w349, "IDs"=w346) -> ("error out"=w350:errorcluster)  [unwired: 4 in, 2 out]
      }
      frame "Cmd_MoveZero" {
        w356 = 0.0 ("element")
        n201 = local read "IDs"() -> (w354:i32[])
        n202 = local read "Calibration"() -> (w355:cluster{dbl, "MicrostepMode":u32}[])
        n203 = Build Array(w356, w356) -> (w357:dbl[])
        n204 = call "PositionControl.vi"("Mode"=PosCtrlOptions."Both X and Y", "error in (no error)"=w359, "Calibration"=w355, "Move to"=w357, "IDs"=w354) -> ("error out"=w358:errorcluster)  [unwired: 3 in, 3 out]
      }
      frame "Cmd_GetPos" {
        n205 = local read "IDs"() -> (w371:i32[])
        n206 = local read "Calibration"() -> (w372:cluster{dbl, "MicrostepMode":u32}[])
        n207 = call "PositionControl.vi"("Mode"=PosCtrlOptions."Read Pos", "error in (no error)"=w374, "Calibration"=w372, "IDs"=w371) -> ("error out"=w373:errorcluster, "Moving?"=→"Moving?":bool, "Position"=w363:sgl[])  [unwired: 4 in, 1 out]
        n208 = Index Array(array=w363, index #1=0 ("index"), index #2=1 ("index")) -> (element #1=w367:sgl, element #2=w366:sgl)
        n209 = local write "X Position"(w367) -> ()
        n210 = local write "Y Position"(w366) -> ()
        n211 = Build Array(w367) -> (w369:sgl[])
        n212 = Build Array(w366) -> (w370:sgl[])
        n213 = Bundle(w369, w370) -> (→"Stage Position":cluster{sgl[], sgl[]})  [unwired: 1 in]
      }
      frame "Cmd_Stop" {
        n214 = local read "IDs"() -> (w377:i32[])
        n215 = for {
          shift-right: [w382] -> w379
          shift-left: w378 -> [w381]
          tunnel: w377 -> [w380] mode=indexing
          n216 = call "command stop.vi"("error in (no error)"=w381, "id"=w380) -> ("error out"=w382:errorcluster)  [unwired: 8 in, 1 out]
        }
      }
      frame "Sync_On" {
        n217 = local read "EdgePt/nPixelMap"() -> (w385:bool)
        n218 = local read "IDs"() -> (w388:i32[])
        n219 = local read "Step Sizes"() -> (w386:sgl[])
        n220 = local read "Calibration"() -> (w387:cluster{dbl, "MicrostepMode":u32}[])
        n221 = call "SetSyncSettings.vi"("Periodic/nPointScan"=w385, "X SyncOut Enabled"=TRUE, "Y SyncOut Enabled"=FALSE, "error in (no error)"=w391, "Calibration"=w387, "Step Sizes(mm)"=w386, "IDs"=w388) -> ("error out"=w390:errorcluster)  [unwired: 3 in, 1 out]
      }
      frame "Sync_Off" {
        n222 = local read "EdgePt/nPixelMap"() -> (w394:bool)
        n223 = local read "IDs"() -> (w397:i32[])
        n224 = local read "Step Sizes"() -> (w395:sgl[])
        n225 = local read "Calibration"() -> (w396:cluster{dbl, "MicrostepMode":u32}[])
        n226 = call "SetSyncSettings.vi"("Periodic/nPointScan"=w394, "X SyncOut Enabled"=FALSE, "Y SyncOut Enabled"=FALSE, "error in (no error)"=w400, "Calibration"=w396, "Step Sizes(mm)"=w395, "IDs"=w397) -> ("error out"=w399:errorcluster)  [unwired: 3 in, 1 out]
      }
      frame "Stop Motion" {
        w402 = TRUE ("Close")
        n227 = local read "IDs"() -> (w404:i32[])
        n228 = for {
          shift-right: [w410] -> w407
          shift-left: w405 -> [w409]
          tunnel: w404 -> [w408] mode=indexing
          n229 = call "command stop.vi"("error in (no error)"=w409, "id"=w408) -> ("error out"=w410:errorcluster)  [unwired: 8 in, 1 out]
        }
        n230 = call "CloseDevices.vi"("error in (no error)"=w407, "Close"=w402, "Ids"=w404) -> ("error out"=w406:errorcluster)  [unwired: 8 in]
        n231 = local write "Moving?"(FALSE ("Moving?")) -> ()
      }
      frame "CloseApplication" {
        w411 = TRUE ("Close")
        n232 = local read "IDs"() -> (w414:i32[])
        n233 = for {
          shift-right: [w420] -> w417
          shift-left: w415 -> [w419]
          tunnel: w414 -> [w418] mode=indexing
          n234 = call "command stop.vi"("error in (no error)"=w419, "id"=w418) -> ("error out"=w420:errorcluster)  [unwired: 8 in, 1 out]
        }
        n235 = call "CloseDevices.vi"("error in (no error)"=w417, "Close"=w411, "Ids"=w414) -> ("error out"=w416:errorcluster)  [unwired: 8 in]
        n236 = local write "Moving?"(FALSE ("Moving?")) -> ()
      }
    }
    n237 = local read "Serial nos"() -> (w5:u32[])
    n238 = call <instrlib>:"Synchronous Latch.vi"("clear"=w13, "set"=w15) -> ("out"=w14:bool)  [unwired: 9 in]
    n239 = Not(x=w14) -> (.not. x?=w7:bool)
    n240 = Greater Than 0?(x=w5) -> (x > 0?=w4:bool[])
    n241 = Or(x=w19, y="Stop Stage") -> (x .or. y?=w16:bool)
    n242 = And Array Elements(Boolean array=w4) -> (logical AND=w3:bool)
    n243 = Select(t=StageOptions."Stop Motion", s=w16, f=w17) -> (s? t:f=w10:T1)
    n244 = And(x=w3, y=w7) -> (x .and. y?=→"Controller Open?":bool)
    n245 = Select(t=StageOptions."CloseApplication", s="Close Stage", f=w10) -> (s? t:f=w11:T1)
    "Stage Status" <- w22
  }
